vi "Main.vi"() -> ()   [LabVIEW 2020, in "Program.lvclass"]
uses:
  Program.lvclass
  ManagerMediator_class/ManagerMediator.lvclass
  C:/Projects/DesignPatterns/Mediator/Mediator_class/Mediator.lvclass
  Programmer_class/Programmer.lvclass
  C:/Projects/DesignPatterns/Mediator/Colleague_class/Colleague.lvclass
  Customer_class/Customer.lvclass
  Tester_class/Tester.lvclass
  Colleague_class/Colleague.lvclass
  Console_class/Console.lvclass
panel:
  out "error out":errorcluster
  out "TextOut":string
  # "The mediator pattern defines an object that encapsulates how a set of objects interact."
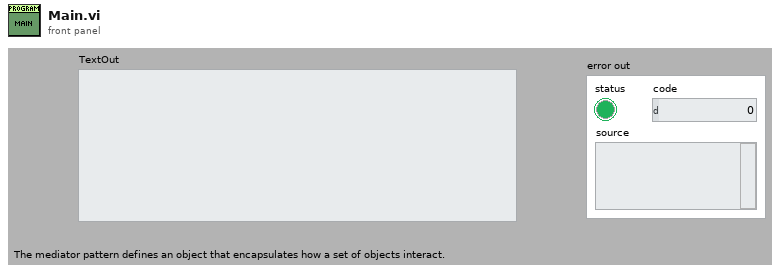
[diagram p1: front panel]
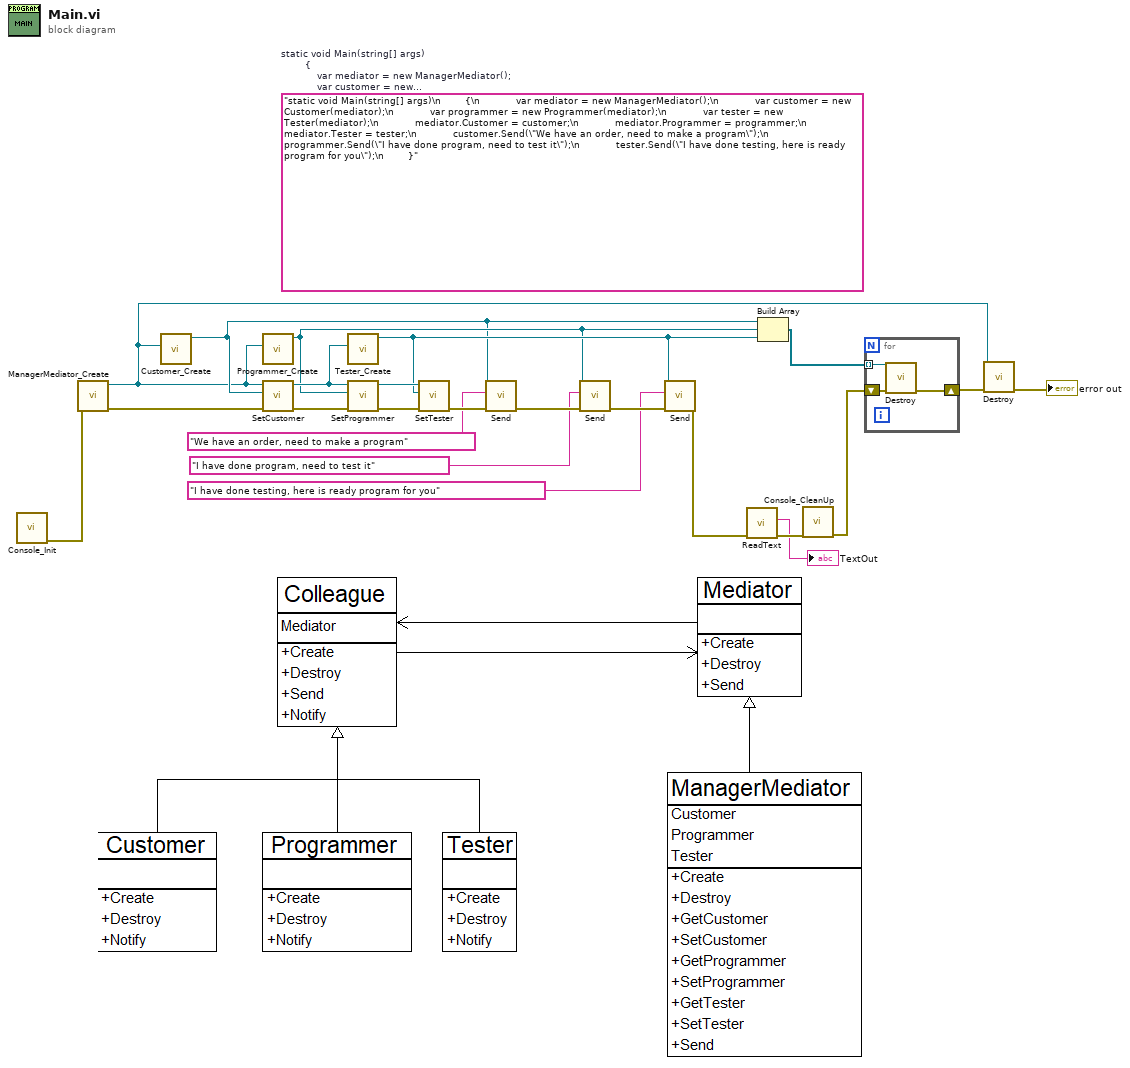
[diagram p0: block diagram]
diagram:
  (unwired) "static void Main(string[] args)\n        {\n            var mediator = new ManagerMediator();\n            var customer = new Customer(mediator);\n            var programmer = new Programmer(mediator);\n            var tester = new Tester(mediator);\n            mediator.Customer = customer;\n            mediator.Programmer = programmer;\n            mediator.Tester = tester;\n            customer.Send(\"We have an order, need to make a program\");\n            programmer.Send(\"I have done program, need to test it\");\n            tester.Send(\"I have done testing, here is ready program for you\");\n        }"  # static void Main(string[] args)         {             var mediator = new ManagerMediator();             var customer = new Customer(mediator);             var programmer = new Programmer(mediator);             var tester = new Tester(mediator);             mediator.Customer = customer;             mediator.Programmer = programmer;             mediator.Tester = tester;             customer.Send("We have an order, need to make a program");             programmer.Send("I have done program, need to test it");             tester.Send("I have done testing, here is ready program for you");         }
  n1 = call "Console_Init.vi"() -> ("Error Out"=w12:errorcluster)  [unwired: 10 in, 1 out]
  n2 = call "ManagerMediator_Create.vi"("Error In"=w12) -> ("Error Out"=w20:errorcluster, "reference out"=w3:refnum<class "ManagerMediator.lvclass">)  [unwired: 9 in]
  n3 = call "Customer_Create.vi"("Mediator"=w3) -> ("reference out"=w7:refnum<class "Customer.lvclass">)  [unwired: 9 in, 1 out]
  n4 = call "Programmer_Create.vi"("Mediator"=w3) -> ("reference out"=w8:refnum<class "Programmer.lvclass">)  [unwired: 9 in, 1 out]
  n5 = call-dynamic "SetCustomer.vi"("Error In"=w20, "Customer"=w7, "reference in"=w3) -> ("Error Out"=w23:errorcluster, "reference in"=w13:refnum<class "ManagerMediator.lvclass">)  [unwired: 7 in]
  n6 = call "Tester_Create.vi"("Mediator"=w13) -> ("reference out"=w9:refnum<class "Tester.lvclass">)  [unwired: 9 in, 1 out]
  n7 = call-dynamic "SetProgrammer.vi"("Error In"=w23, "Programmer"=w8, "reference in"=w13) -> ("Error Out"=w22:errorcluster, "reference in"=w21:refnum<class "ManagerMediator.lvclass">)  [unwired: 7 in]
  n8 = call-dynamic "SetTester.vi"("Error In"=w22, "Tester"=w9, "reference in"=w21) -> ("Error Out"=w19:errorcluster)  [unwired: 7 in, 1 out]
  n9 = call-dynamic "Send.vi"("Error In"=w19, "Message"="We have an order, need to make a program", "reference in"=w7) -> ("Error Out"=w17:errorcluster)  [unwired: 7 in, 1 out]
  n10 = call-dynamic "Send.vi"("Error In"=w17, "Message"="I have done program, need to test it", "reference in"=w8) -> ("Error Out"=w15:errorcluster)  [unwired: 7 in, 1 out]
  n11 = call-dynamic "Send.vi"("Error In"=w15, "Message"="I have done testing, here is ready program for you", "reference in"=w9) -> ("Error Out"=w11:errorcluster)  [unwired: 7 in, 1 out]
  n12 = call "ReadText.vi"("Error In"=w11) -> ("Error Out"=w10:errorcluster, "TextOut"=→"TextOut":string)  [unwired: 9 in]
  n13 = Build Array(w7, w8, w9) -> (w6:refnum<class "Colleague.lvclass">[])
  n14 = call "Console_CleanUp.vi"("Error In"=w10) -> ("Error Out"=w5:errorcluster)  [unwired: 10 in]
  n15 = for {
    tunnel: w6 -> [w26] mode=indexing
    shift-right: [w24] -> w4
    shift-left: w5 -> [w25]
    n16 = call-dynamic "Destroy.vi"("Error In"=w25, "reference in"=w26) -> ("Error Out"=w24:errorcluster)  [unwired: 8 in, 1 out]
  }
  n17 = call-dynamic "Destroy.vi"("Error In"=w4, "reference in"=w3) -> ("Error Out"=→"error out":errorcluster)  [unwired: 8 in, 1 out]
